vi "Write id.vi"(8 "error in (no error)":errorcluster, 10 "id":string, 11 "DSFPlugin in":refnum<class "DSFPlugin.lvclass">) -> (0 "error out":errorcluster, 3 "DSFPlugin out":refnum<class "DSFPlugin.lvclass">)   [LabVIEW 2017, in "DSFPlugin.lvclass"]
uses:
  DSFPlugin.lvclass
  DSFPlugin.lvclass/DSFPlugin.ctl
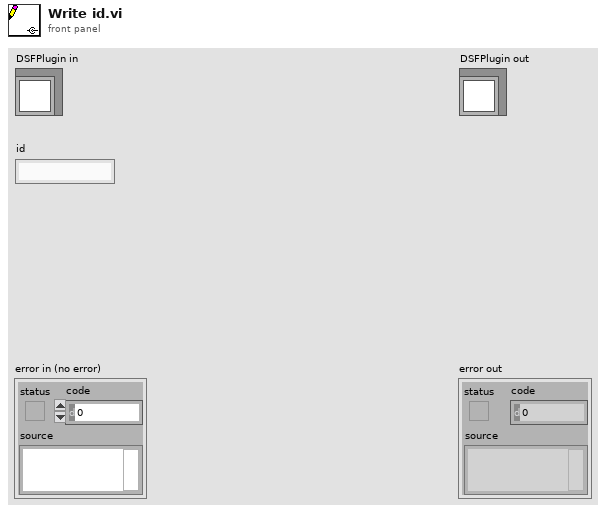
[diagram p1: front panel]
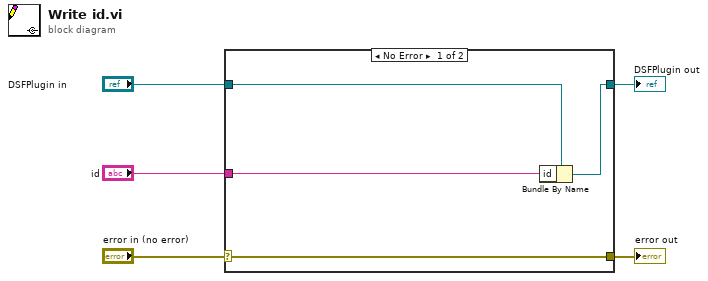
[diagram p0: block diagram]
diagram:
  n1 = case shown="No Error" "error in (no error)" {
    selector: "error in (no error)" -> [w9 w10]
    tunnel: [w9 w10] -> w4
    tunnel: [w7 w11] -> w2
    tunnel: "DSFPlugin in" -> [w8 w11]
    tunnel: "id" -> [w6 _]
    frame No Error {
      n2 = Bundle By Name(cluster=w8, "id"=w6) -> (w7:refnum<class "DSFPlugin.lvclass">)
    }
    frame Error {
    }
  }
  "error out" <- w4
  "DSFPlugin out" <- w2
